vi "AddPassingObject.vi"(0 "object in":refnum<class "Scripting.lvclass">, 1 "PassingThroughObject":string, 2 "PassingThroughObjectName":string, 3 "TerminalName":string, 5 "error in (no error)":errorcluster) -> (14 "object out":refnum<class "Scripting.lvclass">, 19 "error out":errorcluster)   [LabVIEW 2016, in "Scripting.lvclass"]
uses:
  <resource>/Framework/Providers/Open_GDS/ClassProviders/Common/ScriptingFunctions/Scripting.lvclass
  <resource>/Framework/Providers/Open_GDS/ClassProviders/Common/ScriptingFunctions/Scripting_ObjectType.ctl
  <resource>/Framework/Providers/Open_GDS/ClassProviders/Common/ScriptingFunctions/Scripting.lvclass/Scripting.ctl
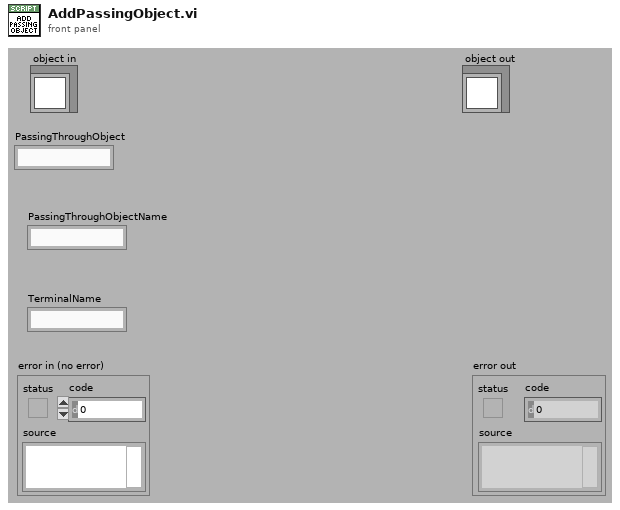
[diagram p1: front panel]
types:
  T1 = typedef "Scripting_ObjectType.ctl" = cluster{"ObjectType":string, "ObjectName":string, "ObjectTerminalName":string}
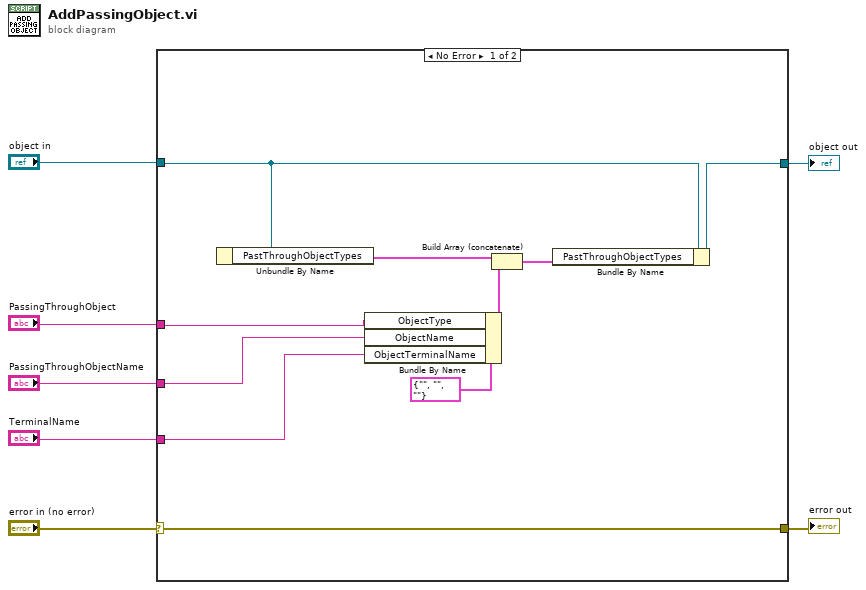
[diagram p0: block diagram]
diagram:
  n1 = case shown="No Error" "error in (no error)" {
    selector: "error in (no error)" -> [w17 w19]
    tunnel: [w17 w19] -> w6
    tunnel: [w15 w18] -> w4
    tunnel: "object in" -> [w16 w18]
    tunnel: "PassingThroughObject" -> [w11 _]
    tunnel: "PassingThroughObjectName" -> [w10 _]
    tunnel: "TerminalName" -> [w9 _]
    frame No Error {
      n2 = Unbundle By Name(w16) -> ("PastThroughObjectTypes"=w14:T1[])
      n3 = Bundle By Name(cluster=T1 {"ObjectType"="", "ObjectName"="", "ObjectTerminalName"=""} ("Cluster"), "ObjectType"=w11, "ObjectName"=w10, "ObjectTerminalName"=w9) -> (w8:T1)
      n4 = Build Array (concatenate)(w14, w8) -> (w13:T1[])
      n5 = Bundle By Name(cluster=w16, "PastThroughObjectTypes"=w13) -> (w15:refnum<class "Scripting.lvclass">)
    }
    frame Error {
    }
  }
  "error out" <- w6
  "object out" <- w4
